vi "GPIB Error Report.vi"(2 "Function":string="Fonction GPIB " caption="Fonction", 3 "Dialog?(F)":bool caption="Boîte de dialogue ? (F)", 4 "Status":bool[](array[boolean])=[FALSE, FALSE, FALSE, FALSE, FALSE, FALSE, FALSE, FALSE, FALSE, FALSE, FALSE, FALSE, FALSE, FALSE, FALSE, FALSE] caption="État", 5 "Address String":string caption="Chaîne d'adresse") -> (0 "Error String":string caption="Chaîne d'erreur", 1 "Status String":string caption="Chaîne d'état")   [LabVIEW 2018]
doc: "Interprète les bits d'état renvoyés par une fonction GPIB et rapporte l'état et toute erreur sous forme de texte. Si Boîte de dialogue est définie à Vrai, le message d'erreur est rapporté dans une boîte de dialogue et l'utilisateur a le choix entre abandonner et continuer."
panel:
  in  "Error strings":string[](array[string])=["EDVR : Erreur lors de la connexion au driver ou au périphérique", "ECIC - La commande nécessite que le contrôleur GPIB soit en charge", "ENOL - L'écriture n'a détecté aucun récepteur", "EADR - Contrôleur GPIB adressé incorrectement", "EARG - Argument(s) non valide(s)", "ESAC - La commande nécessite que le contrôleur GPIB soit le contrôleur du système", "EABO - Opération d'E/S abandonnée", "ENEB - Carte inexistante", "EDMA - Erreur de périphérique DMA détectée", "EBTO - Timeout du bus uP du périphérique DMA", "EOIP - Nouvelle E/S tentée avec une E/S ancienne en cours", "ECAP - Opération non réalisable", "EFSO - Erreur lors d'une opération sur le système de fichiers", "EOWN - Carte partageable en propriété exclusive.", "TIMO - Timeout", "ESTB - Débordement de la file d'attente des octets d'interrogation série (Serial Poll)", "ESRQ - Requête de service bloquée", "ECMD - Commande non reconnue", "", "EBNP - Carte non présente", "EINTRP - Erreur de l'interprète (MacBus)", "", "", "", "", "", "", "", "", "", "NADDR - Aucune entrée d'adresse GPIB", "NSTRG - Aucune chaîne en entrée (écriture)", "NCNT - Aucune entrée de décompte (lecture)", "", "", "", "", "", "", "", "EMOM - Mémoire insuffisante (MacBus)", "EMIM - Mémoire insuffisante (MacBus)", "", "", "", "", "", "", "", "", "ECOMM - Échec au niveau des protocoles SCSI (MacBus)", "", "", "", "", "", "", "", "", "", "", "EPAR - Le système n'a pas pu allouer la mémoire nécessaire", "EORN - Le système a provoqué l'abandon de la connexion au réseau", "EOFL - Débordement du buffer d'entrées du port série", "EFRM - La connexion au réseau n'est pas encore établie", "SPTMO - Timeout du port série, aucun octet reçu."] caption="Chaînes d'erreur"
  in  "Status bit strings":string[](array[string])=["DCAS - Réinitialisation du périphérique", "DTAS - Déclenchement du périphérique", "LACS - État actif du récepteur", "TACS - État actif de l'émetteur", "ATN - Attention activée", "CIC - Contrôleur en charge", "REM - État déporté", "LOK - État Lockout", "CMPL - Opération terminée", "", "", "", "SRQI - Requête de service détectée pendant que le contrôleur était en charge", "END - EOI ou EOS détectée", "TIMO - Timeout", "ERR - Erreur détectée"] caption="Chaînes de bit d'état"
  # "Ce VI est inclus pour des raisons de compatibilité avec des versions antérieures. \nIl n'est pas utilisé dans l'exemple."
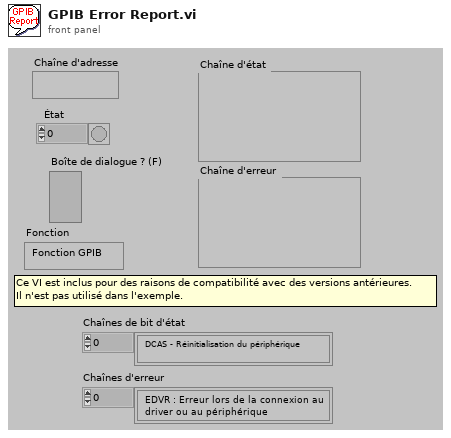
[diagram p1: front panel]
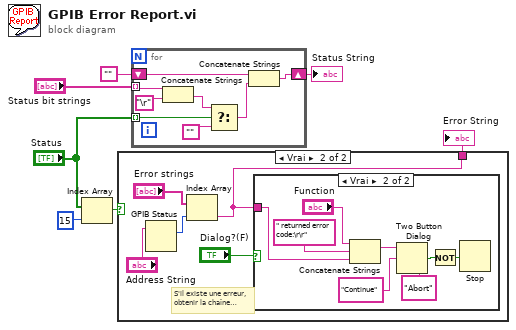
[diagram p0: block diagram]
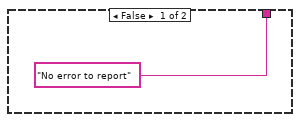
[diagram p2: hidden frame]
diagram:
  n1 = Index Array(array="Status", index=15) -> (element=w2:bool)
  n2 = case shown="Vrai" w2 {
    tunnel: ["No error to report" w9] -> w1
    frame False {
    }
    frame True {
      # "S'il existe une erreur, obtenir la chaîne d'erreur"
      n3 = GPIB Status(0:"Address String") -> (3:w11:i16)  [unwired: 1 in, 3 out]
      n4 = Index Array(array="Error strings", index=w11) -> (element=w9:string)
      n5 = case shown="Vrai" "Dialog?(F)" {
        tunnel: w9 -> [_ w14]
        frame False {
        }
        frame True {
          n6 = Concatenate Strings("Function", " returned error code:\r\r", w14) -> (w20:string)
          n7 = Two Button Dialog(message=w20, 1:"Abort", 2:"Continue") -> (T button?=w17:bool)
          n8 = Not(x=w17) -> (.not. x?=w16:bool)
          n9 = Stop(stop? (T)=w16) -> ()
        }
      }
    }
  }
  "Error String" <- w1
  n10 = for {
    shift-right: [w22] -> w5
    shift-left: "" -> [w24]
    tunnel: "Status" -> [w27] mode=indexing
    tunnel: "Status bit strings" -> [w29] mode=indexing
    n11 = Concatenate Strings(w29, "\r") -> (w26:string)
    n12 = Select(t=w26, s=w27, f="") -> (s? t:f=w23:string)
    n13 = Concatenate Strings(w24, w23) -> (w22:string)
  }
  "Status String" <- w5
